vi "Gill_parse_response.vi"(0 "Address letter":string, 1 "Stripped Gill response":string, 2 "GILL TYPE NO.":i32) -> (4 "Numerics":dbl[](array[numeric]) format="%.2f", 5 "Status":u8, 6 "Error notes":string)   [LabVIEW 2014]
panel:
  out "Type\nModel 2":u8
  out "Type\nModel":u8
  in  "Status Messages":string[](array[string])=["", "Transducer Pair 1 failed", "Transducer Pair 2 failed", "Transducers 1 & 2 failed", "Non-volatile Checksum error", "Volatile memory checksum error", "System gain at maximum", "Marginal system gain condition", "Measurement average building", "Heating operational", "Heating OK but under power", "Heating tripped", "Temperature sensor fault", "Heating OK but over power"]
  in  "Status Codes":u8[](array[numeric])=[0, 1, 2, 4, 8, 9, 10, 50, 51, 60, 61, 62, 63, 64]
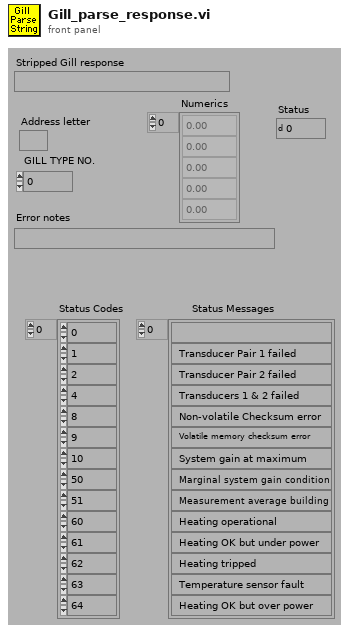
[diagram p1: front panel]
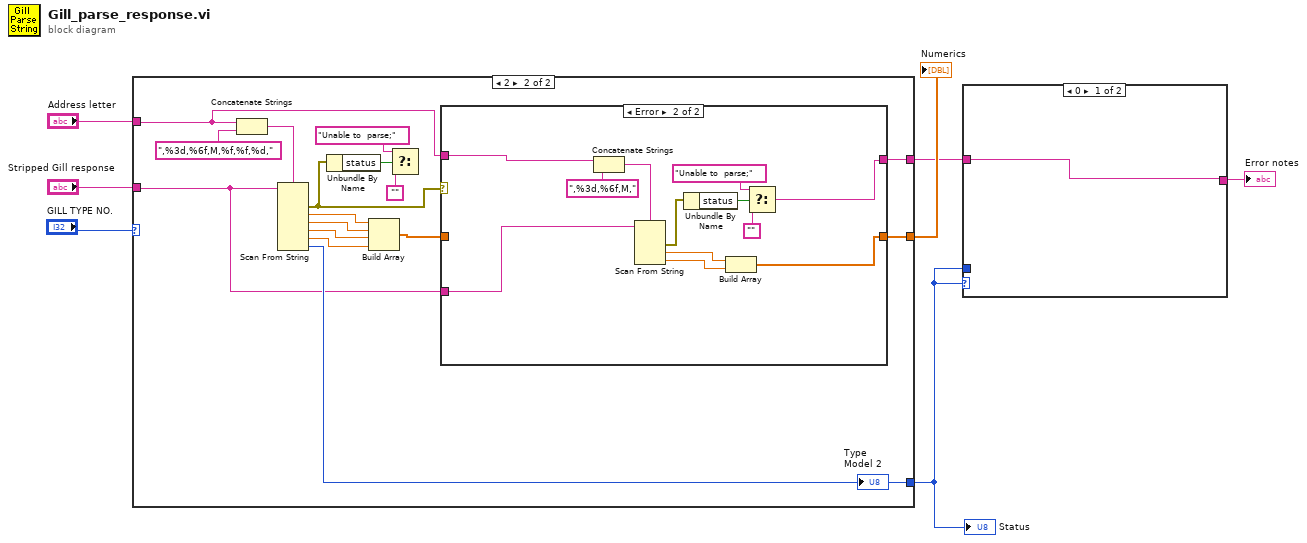
[diagram p0: block diagram]
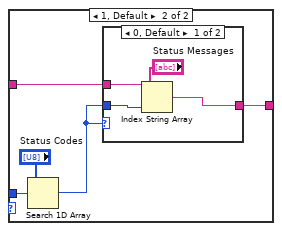
[diagram p2: hidden frame]
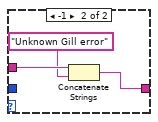
[diagram p3: hidden frame]
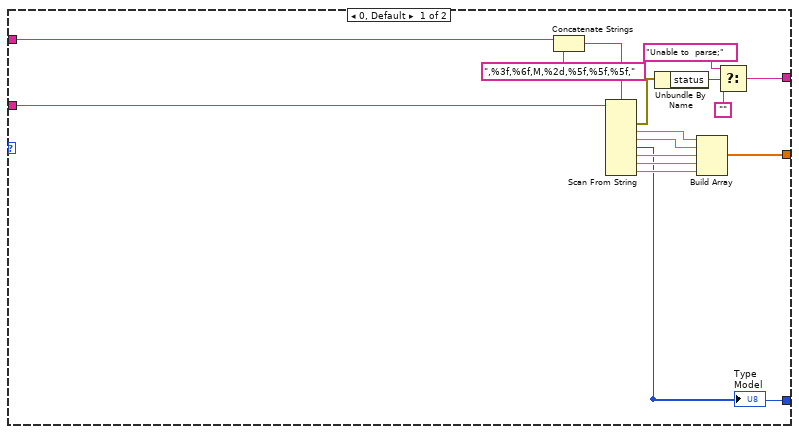
[diagram p4: hidden frame]
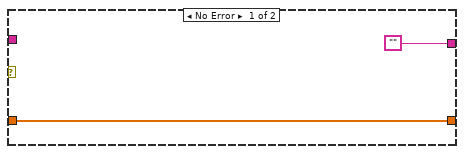
[diagram p5: hidden frame]
diagram:
  n1 = case shown="2" "GILL TYPE NO." {
    tunnel: "Stripped Gill response" -> [w23 w24]
    tunnel: "Address letter" -> [w22 w25]
    tunnel: [w15 w26] -> w5
    tunnel: [w10 w28] -> w3
    tunnel: [w8 w30] -> w1
    frame 0, Default {
      n2 = Concatenate Strings(w22, ",%3f,%6f,M,%2d,%5f,%5f,%5f,") -> (w21:string)
      n3 = Scan From String(format string=w21, input string=w23) -> (error out=w13:errorcluster, output 1=w16:dbl, output 2=w17:dbl, output 3=w8:u8, output 4=w18:dbl, output 5=w19:dbl, output 6=w20:dbl)  [unwired: 2 in, 8 out]
      "Type\nModel" <- w8
      n4 = Unbundle By Name(w13) -> ("status"=w12:bool)
      n5 = Build Array(w16, w17, w18, w19, w20) -> (w15:dbl[])
      n6 = Select(t="Unable to  parse;", s=w12, f="") -> (s? t:f=w10:string)
    }
    frame 2 {
      n7 = Concatenate Strings(w25, ",%3d,%6f,M,%f,%f,%d,") -> (w31:string)
      n8 = Scan From String(format string=w31, input string=w24) -> (error out=w29:errorcluster, output 1=w38:dbl, output 2=w39:dbl, output 3=w33:dbl, output 4=w32:dbl, output 5=w30:u8)  [unwired: 2 in, 7 out]
      "Type\nModel 2" <- w30
      n9 = Unbundle By Name(w29) -> ("status"=w36:bool)
      n10 = Build Array(w38, w39, w33, w32) -> (w27:dbl[])
      n11 = Select(t="Unable to  parse;", s=w36, f="") -> ()  [unwired: 1 out]
      n12 = case shown="Error" w29 {
        tunnel: ["" w43] -> w28
        tunnel: w27 -> [w40 _]
        tunnel: [w40 w42] -> w26
        tunnel: w25 -> [_ w45]
        tunnel: w24 -> [_ w44]
        frame No Error {
        }
        frame Error {
          n13 = Concatenate Strings(w45, ",%3d,%6f,M,") -> (w52:string)
          n14 = Scan From String(format string=w52, input string=w44) -> (error out=w53:errorcluster, output 1=w47:dbl, output 2=w46:dbl)  [unwired: 2 in, 4 out]
          n15 = Unbundle By Name(w53) -> ("status"=w49:bool)
          n16 = Build Array(w47, w46) -> (w42:dbl[])
          n17 = Select(t="Unable to  parse;", s=w49, f="") -> (s? t:f=w43:string)
        }
      }
    }
  }
  "Numerics" <- w5
  "Status" <- w1
  n18 = case shown="0" w1 {
    tunnel: w1 -> [_ w58]
    tunnel: w3 -> [w54 w57]
    tunnel: [w54 w56] -> w2
    frame 0 {
    }
    frame 1, Default {
      n19 = Search 1D Array(1D array="Status Codes", element=w58) -> (index of element=w55:i32)  [unwired: 1 out]
      n20 = case shown="0, Default" w55 {
        tunnel: w57 -> [w63 w66]
        tunnel: [w62 w65] -> w56
        tunnel: w55 -> [w60 _]
        frame 0, Default {
          n21 = Index String Array(1:w60, 2:"Status Messages", 3:w63) -> (0:w62:string)
        }
        frame -1 {
          n22 = Concatenate Strings(w66, "Unknown Gill error" ("Substring")) -> (w65:string)
        }
      }
    }
  }
  "Error notes" <- w2
